vi "MV3D RGBD Get Calib Info.vi"(9 "pstCalibInfo":T1, 10 "nCoordinateType":u32, 11 "handle":u32) -> (1 "pstCalibInfo out":T1, 2 "function return":i32, 3 "handle out":u32)   [LabVIEW 2015, in "Mv3dRgbd.lvlib"]
doc: "MV3D_RGBD_API MV3D_RGBD_STATUS MV3D_RGBD_GetCalibInfo(HANDLE handle, uint32_t nCoordinateType, MV3D_RGBD_CALIB_INFO *pstCalibInfo);"
uses:
  <userlib>/Mv3dRgbd/Mv3dRgbd.lvlib
  <userlib>/Mv3dRgbd/Mv3dRgbd.dll
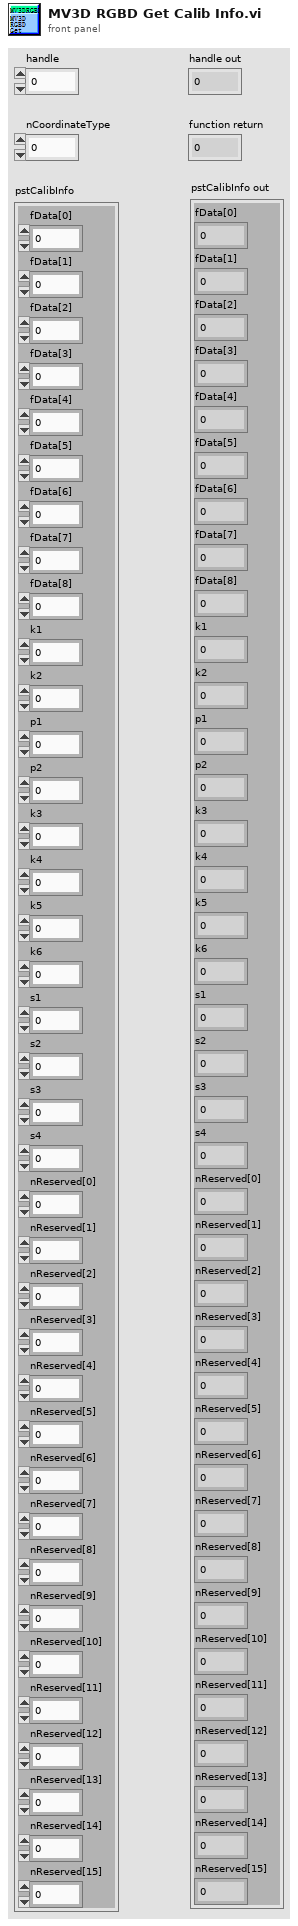
[diagram p1: front panel]
types:
  T1 = cluster{"fData[0]":sgl, "fData[1]":sgl, "fData[2]":sgl, "fData[3]":sgl, "fData[4]":sgl, "fData[5]":sgl, "fData[6]":sgl, "fData[7]":sgl, "fData[8]":sgl, "k1":sgl, "k2":sgl, "p1":sgl, "p2":sgl, "k3":sgl, "k4":sgl, "k5":sgl, "k6":sgl, "s1":sgl, "s2":sgl, "s3":sgl, "s4":sgl, "nReserved[0]":u8, "nReserved[1]":u8, "nReserved[2]":u8, "nReserved[3]":u8, "nReserved[4]":u8, "nReserved[5]":u8, "nReserved[6]":u8, "nReserved[7]":u8, "nReserved[8]":u8, "nReserved[9]":u8, "nReserved[10]":u8, "nReserved[11]":u8, "nReserved[12]":u8, "nReserved[13]":u8, "nReserved[14]":u8, "nReserved[15]":u8}
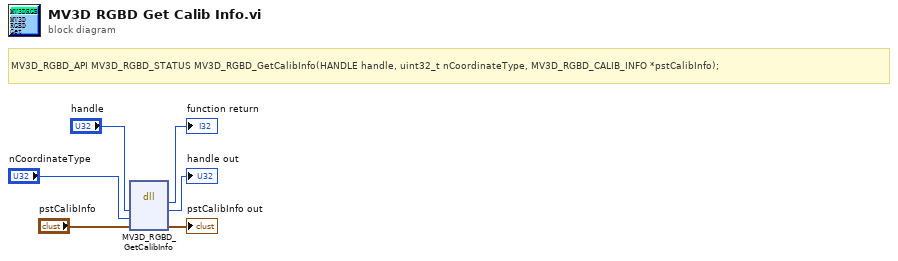
[diagram p0: block diagram]
diagram:
  # "MV3D_RGBD_API MV3D_RGBD_STATUS MV3D_RGBD_GetCalibInfo(HANDLE handle, uint32_t nCoordinateType, MV3D_RGBD_CALIB_INFO *pstCalibInfo);"
  n1 = dll-call lib="C:/Program Files (x86)/National Instruments/LabVIEW 2015/user.lib/Mv3dRgbd/Mv3dRgbd.*" fn="MV3D_RGBD_GetCalibInfo"("handle"="handle", "nCoordinateType"="nCoordinateType", "pstCalibInfo"="pstCalibInfo") -> (→"function return":i32, "handle"=→"handle out":u32, "pstCalibInfo"=→"pstCalibInfo out":T1)  [unwired: 4 in, 2 out]
